vi "Write Start ConfigDir.vi"(8 "error in (no error)":errorcluster, 10 "Start ConfigDir":path=path "C:/Users/user/Desktop/test/ConfigDir", 11 "HIJ Multiple Cams App Demo in":refnum<class "HIJ 4 Alignment Cams App.lvclass">) -> (0 "error out":errorcluster, 3 "HIJ Multiple Cams App Demo out":refnum<class "HIJ 4 Alignment Cams App.lvclass">)   [LabVIEW 2014, in "HIJ 4 Alignment Cams App.lvlib" / "HIJ 4 Alignment Cams App.lvclass"]
uses:
  HIJ 4 Alignment Cams App.lvclass
  HIJ 4 Alignment Cams App.lvclass/HIJ 4 Alignment Cams App.ctl
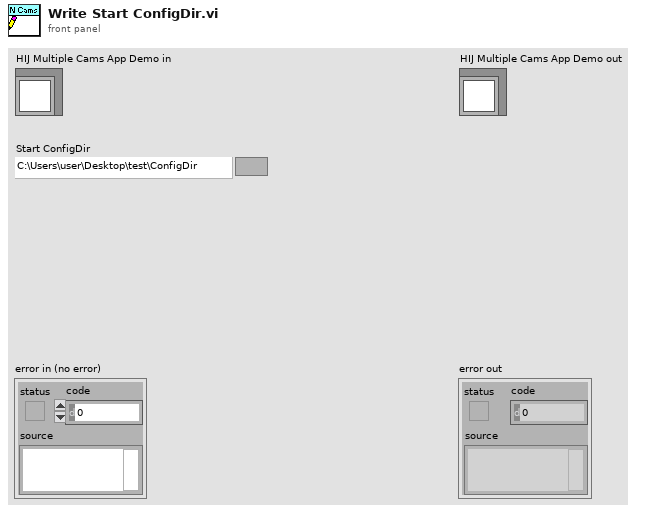
[diagram p1: front panel]
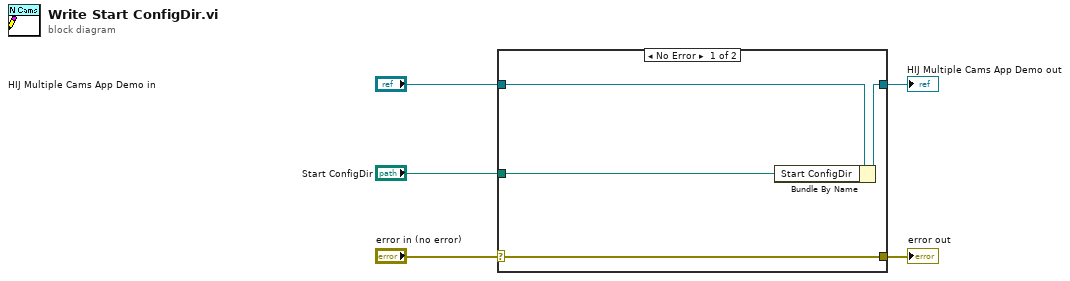
[diagram p0: block diagram]
diagram:
  n1 = case shown="No Error" "error in (no error)" {
    selector: "error in (no error)" -> [w9 w10]
    tunnel: [w9 w10] -> w4
    tunnel: [w7 w11] -> w2
    tunnel: "HIJ Multiple Cams App Demo in" -> [w8 w11]
    tunnel: "Start ConfigDir" -> [w6 _]
    frame No Error {
      n2 = Bundle By Name(cluster=w8, "Start ConfigDir"=w6) -> (w7:refnum<class "HIJ 4 Alignment Cams App.lvclass">)
    }
    frame Error {
    }
  }
  "error out" <- w4
  "HIJ Multiple Cams App Demo out" <- w2
